vi "Get Pose by Name.vi"(8 "error in (no error)":errorcluster, 10 "name":string, 11 "serial arm in":refnum<class "NI_Robotics_Serial Robot Arm.lvclass">) -> (0 "error out":errorcluster, 2 "serial arm pose":T1, 3 "serial arm out":refnum<class "NI_Robotics_Serial Robot Arm.lvclass">)   [LabVIEW 2017, in "NI_Robotics_Serial Robot Arm.lvclass"]
doc: "Returns the joint angles that make up the <B>serial arm pose</B> of the name you specify."
uses:
  <vilib>/robotics/Kinematics/Robot/NI_Robotics_Serial Robot Arm.lvclass
  <vilib>/robotics/Kinematics/Robot/Robot Pose.ctl
  <vilib>/robotics/Kinematics/Robot/NI_Robotics_Serial Robot Arm.lvclass/NI_Robotics_Serial Robot Arm.ctl
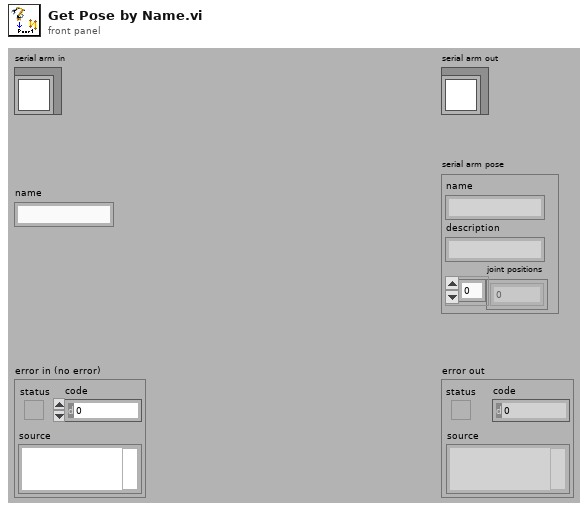
[diagram p1: front panel]
types:
  T1 = typedef "NI_Robotics_Serial Robot Arm.lvclass/Robot Pose.ctl" = cluster{"name":string, "description":string, "joint positions":dbl[]}
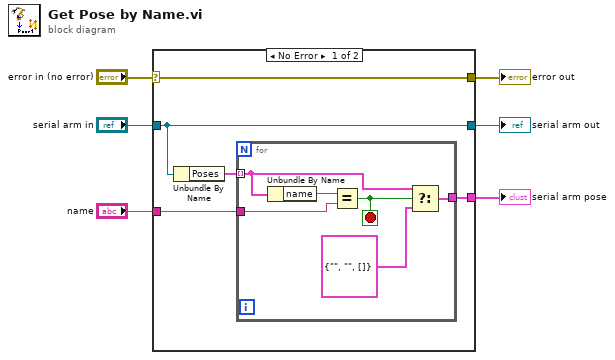
[diagram p0: block diagram]
diagram:
  n1 = case shown="No Error" "error in (no error)" {
    selector: "error in (no error)" -> [w11 w18]
    tunnel: [w11 w18] -> w5
    tunnel: [w10 w19] -> w3
    tunnel: "serial arm in" -> [w10 w19]
    tunnel: [w7 _] -> w1
    tunnel: "name" -> [w8 _]
    frame No Error {
      n2 = Unbundle By Name(w10) -> ("Poses"=w9:T1[])
      n3 = for {
        tunnel: w9 -> [w14] mode=indexing
        tunnel: w8 -> [w16]
        tunnel: [w15] -> w7
        stop <- w12 stop-if-true
        n4 = Unbundle By Name(w14) -> ("name"=w17:string)
        n5 = Equal?(x=w17, y=w16) -> (x = y?=w12:bool)
        n6 = Select(t=w14, s=w12, f=T1 {"name"="", "description"="", "joint positions"=[]}) -> (s? t:f=w15:T1)
      }
    }
    frame Error {
    }
  }
  "error out" <- w5
  "serial arm out" <- w3
  "serial arm pose" <- w1
